vi "pessimize_error_one.vi"(0 "Parameters":T3, 7 "Start point":dbl[](array[numeric]) format="%#_3p", 12 "Pessimize fun info":T4 {"Point selector"."Light number" min=0 max=5}) -> (4 "Pose bias":dbl[](array[numeric]) format="%#_3p", 6 "Error vector":dbl[](array[numeric]) format="%#_3p", 8 "f(X)":dbl, 10 "X at maximum":dbl[](array[numeric]) format="%#_3p", 15 "error out":errorcluster)   [LabVIEW 2013]
uses:
  pessimize_objective_fun_info.ctl
  calibration/point_selector.ctl
  ui_override_opts.ctl
  <vilib>/Analysis/Matrix/Datatypes/RealMatrix.ctl
  <vilib>/gmath/NumericalOptimization/stopping criteria.ctl
  <vilib>/gmath/NumericalOptimization/cno_bounds.ctl
  <vilib>/gmath/NumericalOptimization/Downhill Simplex.vi
  <vilib>/gmath/NI_Gmath.lvlib
  <vilib>/Analysis/Matrix/NI_Matrix.lvlib
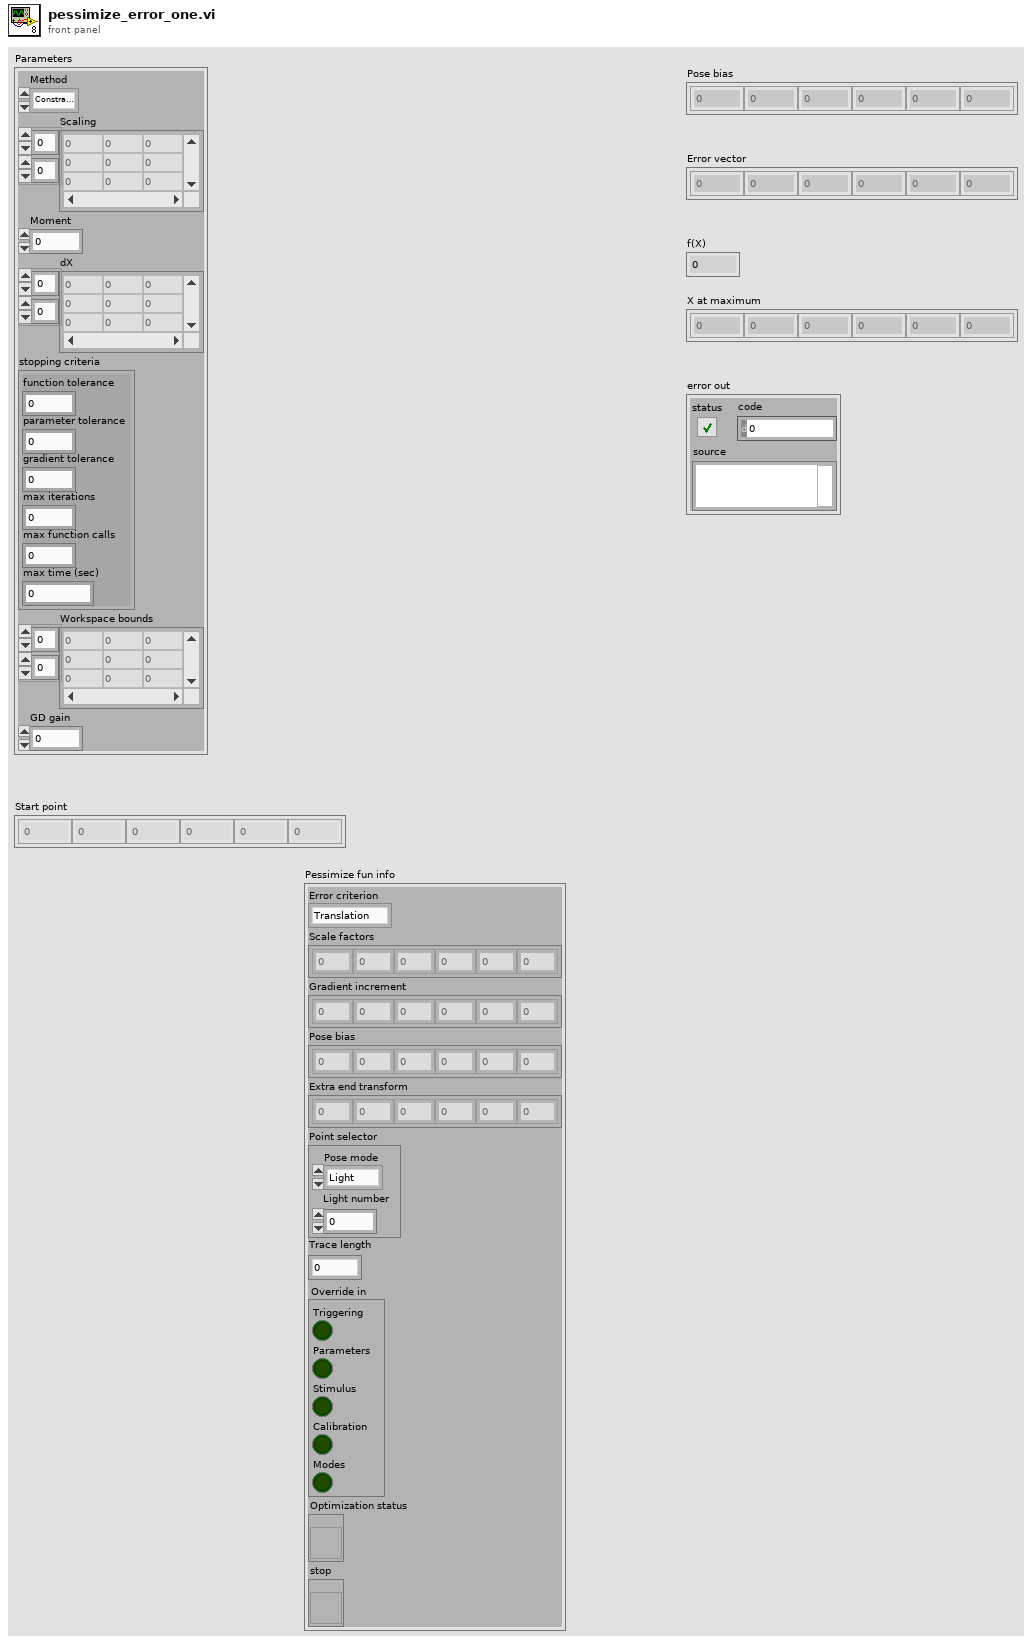
[diagram p1: front panel]
types:
  T1 = typedef "NI_Matrix.lvlib/RealMatrix.ctl" = dbl[][]
  T2 = typedef "NI_Gmath.lvlib/stopping criteria.ctl" = cluster{"function tolerance":dbl, "parameter tolerance":dbl, "max iterations":i32, "max function calls":i32, "gradient tolerance":dbl, "max time (sec)":dbl}
  T3 = cluster{"Method":enum16{"Constrained NL", "Simplex", "Gradient descent"}, "Scaling":T1, "Moment":dbl, "dX":T1, "stopping criteria":T2, "Workspace bounds":T1, "GD gain":dbl}
  T4 = typedef "pessimize_objective_fun_info.ctl" = cluster{"Error criterion":enum16{"Translation", "Orientation", "Moment"}, "Scale factors":dbl[], "Gradient increment":dbl[], "Pose bias":dbl[], "Extra end transform":dbl[], "Point selector":T5, "Trace length":dbl, "Override in":T6, "Optimization status":refnum<vi>, "stop":refnum<vi>}
  T5 = typedef "point_selector.ctl" = cluster{"Pose mode":enum16{"Light", "Handle", "Output"}, "Light number":i32}
  T6 = typedef "ui_override_opts.ctl" = cluster{"Triggering":bool, "Parameters":bool, "Stimulus":bool, "Calibration":bool, "Modes":bool}
  T7 = enum16{"Constrained NL", "Simplex", "Gradient descent"}
  T8 = typedef "NI_Gmath.lvlib/cno_bounds.ctl" = cluster{"X minimum":dbl[], "X maximum":dbl[], "inequality constraint minimum":dbl[], "inequality constraint maximum":dbl[]}
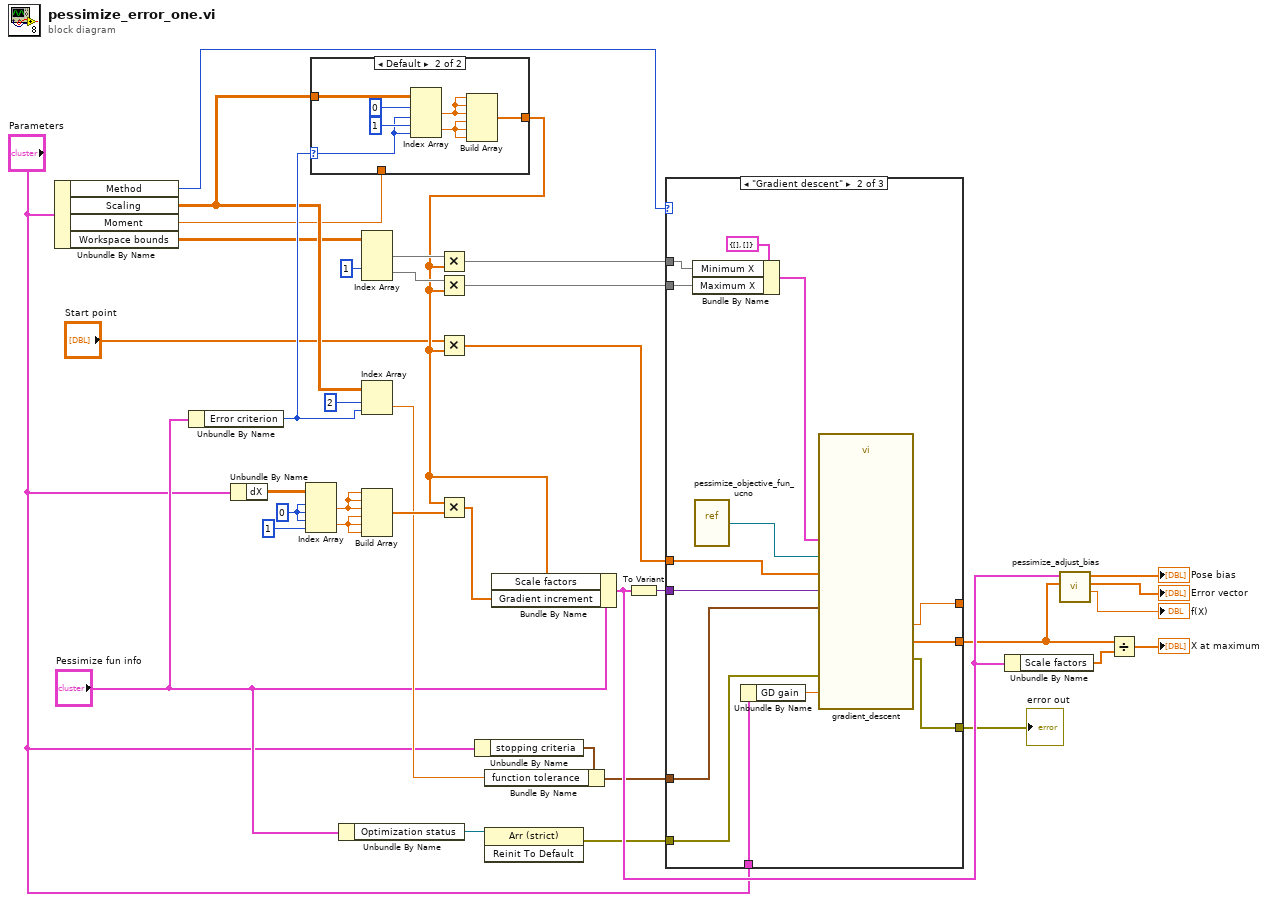
[diagram p0: block diagram]
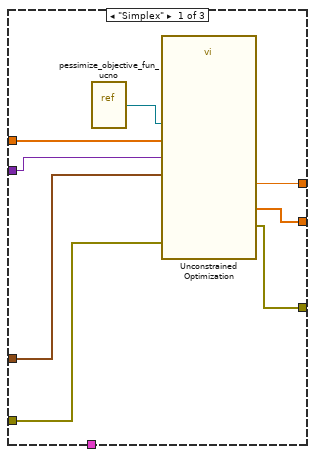
[diagram p2: hidden frame]
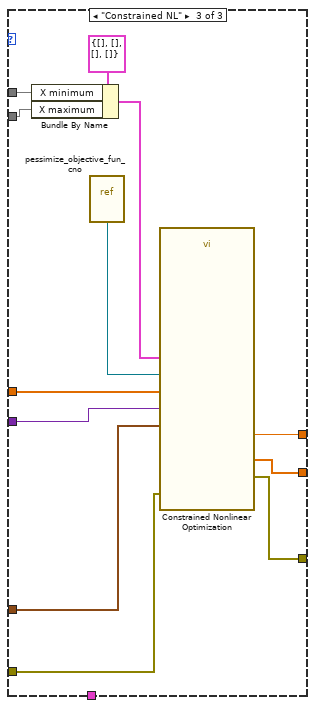
[diagram p3: hidden frame]
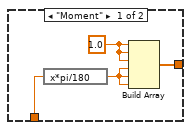
[diagram p4: hidden frame]
diagram:
  w31 = 0 ("disabled index (row)")
  n1 = Unbundle By Name("Parameters") -> ("Method"=w12:T7, "Scaling"=w11:T1, "Moment"=w10:dbl, "Workspace bounds"=w9:T1)
  n2 = Unbundle By Name("Pessimize fun info") -> ("Error criterion"=w37:enum16{"Translation", "Orientation", "Moment"})
  n3 = Unbundle By Name("Parameters") -> ("dX"=w5:T1)
  n4 = Index Array(array=w5, index (row) #1=w31, index (col) #1=w31, index (row) #2=w31, index (col) #2=1 ("disabled index (row)")) -> (element #1=w28:dbl, element #2=w27:dbl)
  n5 = case shown="Default" w37 {
    selector: w37 -> [_ w42]
    tunnel: w11 -> [_ w46]
    tunnel: [w39 w43] -> w8
    tunnel: w10 -> [w38 _]
    frame "Moment" {
      w41 = 1.0 ("element")
      n6 = expression code="x*pi/180"(w38) -> (w40:dbl)
      n7 = Build Array(w41, w41, w41, w40, w40, w40) -> (w39:dbl[])
    }
    frame Default {
      n8 = Index Array(array=w46, index (row) #1=0 ("disabled index (row)"), index (col) #1=w42, index (row) #2=1 ("disabled index (row)"), index (col) #2=w42) -> (element #1=w45:dbl, element #2=w44:dbl)
      n9 = Build Array(w45, w45, w45, w44, w44, w44) -> (w43:dbl[])
    }
  }
  n10 = Unbundle By Name("Pessimize fun info") -> ("Optimization status"=w13:refnum<vi>)
  n11 = Index Array(array=w9, index (row) #2=1 ("index (row)")) -> (element #1=w20:dbl[], element #2=w19:dbl[])  [unwired: 3 in]
  n12 = Index Array(array=w11, index (row)=2 ("disabled index (row)"), index (col)=w37) -> (element=w23:dbl)
  n13 = Build Array(w28, w28, w28, w27, w27, w27) -> (w29:dbl[])
  n14 = Multiply(x=w20, y=w8) -> (x*y=w22:dbl[])
  n15 = Multiply(x=w19, y=w8) -> (x*y=w21:dbl[])
  n16 = Multiply(x="Start point", y=w8) -> (x*y=w26:dbl[])
  n17 = Multiply(x=w8, y=w29) -> (x*y=w36:dbl[])
  n18 = Unbundle By Name("Parameters") -> ("stopping criteria"=w7:T2)
  n19 = Bundle By Name(cluster=w7, "function tolerance"=w23) -> (w18:T2)
  n20 = invoke on="Invoke Node" class="Arr (strict)" method="Reinit To Default"(reference=w13) -> (error out=w24:errorcluster)  [unwired: 2 in, 2 out]
  n21 = Bundle By Name(cluster="Pessimize fun info", "Scale factors"=w8, "Gradient increment"=w36) -> (w35:T4)
  n22 = To Variant(anything=w35) -> (Variant=w17:variant)
  n23 = case shown="\"Gradient descent\"" w12 {
    tunnel: [w56 w60 w80] -> w32
    tunnel: w17 -> [w53 w68 w79]
    tunnel: w18 -> [w55 w70 w78]
    tunnel: w21 -> [_ w62 w77]
    tunnel: w22 -> [_ w63 w76]
    tunnel: w26 -> [w54 w69 w74]
    tunnel: w24 -> [w52 w67 w73]
    tunnel: [w51 w66 w72] -> w25
    tunnel: [w49 w59 w71] -> _
    tunnel: "Parameters" -> [_ w58 _]
    frame "Simplex" {
      n24 = vi-ref "pessimize_objective_fun_ucno.vi"() -> (w50:refnum<vi>)
      n25 = call-poly <vilib>:"Unconstrained Optimization.vi"("function data"=w53, "objective function"=w50, "error in (no error)"=w52, "stopping criteria"=w55, "start"=w54) -> ("error out"=w51:errorcluster, "f(minimum)"=w49:dbl, "minimum"=w56:dbl[])  [unwired: 3 in, 1 out]
    }
    frame "Gradient descent" {
      n26 = Bundle By Name(cluster=cluster{"Minimum X":dbl[], "Maximum X":dbl[]} {"Minimum X"=[], "Maximum X"=[]} ("Bounds"), "Minimum X"=w63, "Maximum X"=w62) -> (w61:cluster{"Minimum X":dbl[], "Maximum X":dbl[]})
      n27 = vi-ref "pessimize_objective_fun_ucno.vi"() -> (w65:refnum<vi>)
      n28 = Unbundle By Name(w58) -> ("GD gain"=w57:dbl)
      n29 = call "gradient_descent.vi"("Gain"=w57, "function data"=w68, "Bounds"=w61, "objective function"=w65, "error in"=w67, "stopping criteria"=w70, "start"=w69) -> ("error out"=w66:errorcluster, "f(X) min"=w59:dbl, "minimum"=w60:dbl[])  [unwired: 2 in]
    }
    frame "Constrained NL" {
      n30 = Bundle By Name(cluster=T8 {"X minimum"=[], "X maximum"=[], "inequality constraint minimum"=[], "inequality constraint maximum"=[]} ("bounds"), "X minimum"=w76, "X maximum"=w77) -> (w81:T8)
      n31 = vi-ref "pessimize_objective_fun_cno.vi"() -> (w75:refnum<vi>)
      n32 = call <vilib>:"Constrained Nonlinear Optimization.vi"("start"=w74, "objective and constraint function"=w75, "function data"=w79, "bounds"=w81, "error in (no error)"=w73, "stopping criteria"=w78) -> ("minimum"=w80:dbl[], "f(minimum)"=w71:dbl, "error out"=w72:errorcluster)  [unwired: 5 in, 2 out]
    }
  }
  "error out" <- w25
  n33 = Unbundle By Name(w35) -> ("Scale factors"=w33:dbl[])
  n34 = call "pessimize_adjust_bias.vi"("X at maximum"=w32, "Pessimize fun info"=w35) -> ("f(X)"=→"f(X)":dbl, "Error vector"=→"Error vector":dbl[], "Pose bias"=→"Pose bias":dbl[])  [unwired: 7 in]
  n35 = Divide(x=w32, y=w33) -> (x/y=→"X at maximum":dbl[])
